vi "NI VeriStand - Ref Constants.vi"() -> ()   [LabVIEW 2020, in "Custom Device Utility Library.lvlib"]
doc: "Creates a global variable that you can use as a reference to the root item in the custom device hierarchy, or as an invalid reference."
uses:
  <vilib>/NI VeriStand/Custom Device Tools/Custom Device Utility Library/Custom Device Utility Library.lvlib
  <vilib>/NI VeriStand/Custom Device API/Custom Device Item Ref.ctl
  <vilib>/NI VeriStand/Custom Device API/Custom Device API.lvlib
panel:
  in  "Root Item Ref":T1 format="%.0x"
  in  "Invalid Ref":T1=18446744073709551615 format="%.0x"
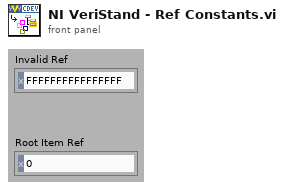
[diagram p1: front panel]
types:
  T1 = typedef "Custom Device API.lvlib/Custom Device Item Ref.ctl" = u64
diagram:
